vi "Gasteiler Korrektur.vi"() -> ()   [LabVIEW 2020, in "Linearisierung v2.lvlib" / "Gasteiler.lvlib"]
uses:
  Gasteiler.lvlib
  Visualisierungs Elemente/Button.ctl
  Aktion FGV Gasteiler Korrektur.ctl
  Allgemein/allgemeine Sub-VIs.lvlib
panel:
  in  "Aktiv":bool
  out "Gültig":bool
  in  "Gültigkeit bis":timestamp[](array[timestamp]) format="%<%Y/%m/%d>T"
  in  "Gasteiler":enum16{"1", "2", "3", "4", "5"}(ring)
  in  "Seriennummer":string[](array[string])
  in  "Stopp":T1
  in  "Speichern":T1
  in  "Abweichung":sgl[][](array[numeric]) format="%#_5g"
  # "Gasteiler Abweichung"
  # "100%"
  # "90%"
  # "80%"
  # "70%"
  # "60%"
  # "50%"
  # "40%"
  # "30%"
  # "20%"
  # "10%"
  # "0%"
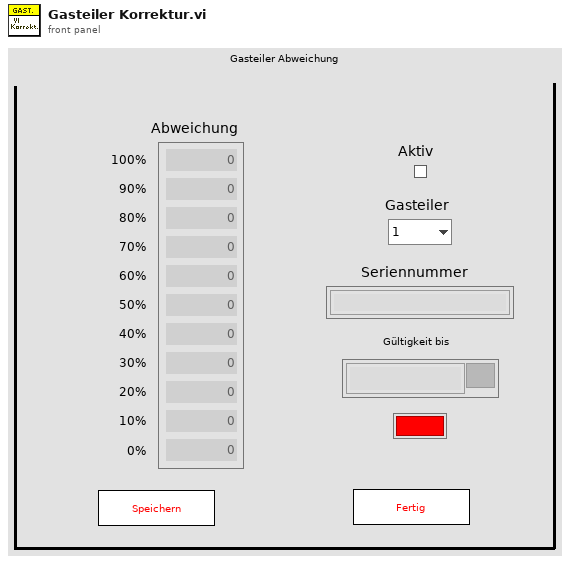
[diagram p1: front panel]
types:
  T1 = typedef "Button.ctl" = bool
  T2 = typedef "Linearisierung v2.lvlib/Gasteiler.lvlib/Aktion FGV Gasteiler Korrektur.ctl" = enum16{"lesen", "schreiben", "laden", "speichern", "B-nr und Gültig", "Gasteilernr.", "Vereinzeln", "aktiv"}
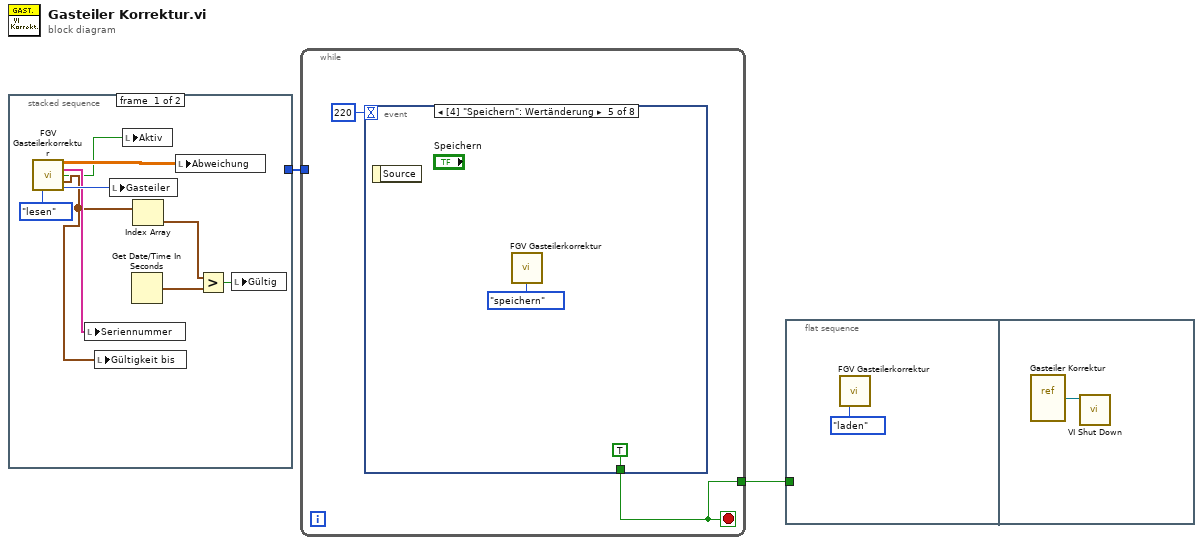
[diagram p0: block diagram]
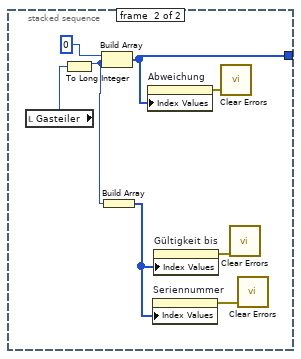
[diagram p2: hidden frame]
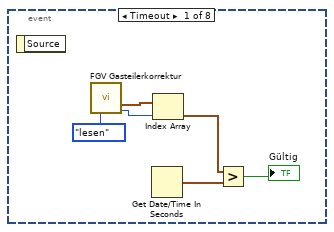
[diagram p3: hidden frame]
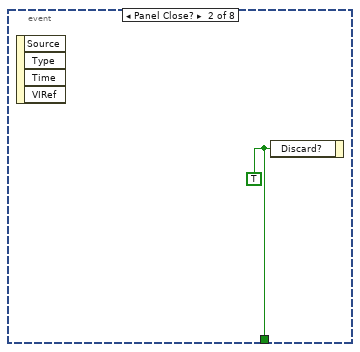
[diagram p4: hidden frame]
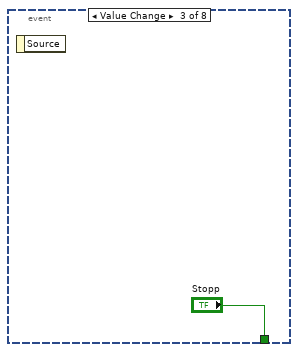
[diagram p5: hidden frame]
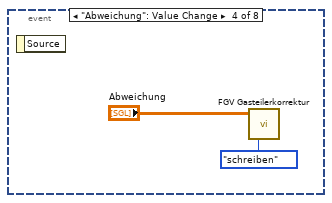
[diagram p6: hidden frame]
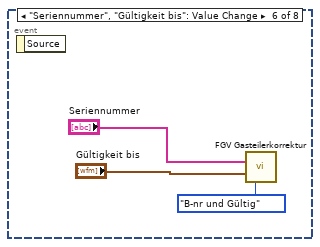
[diagram p7: hidden frame]
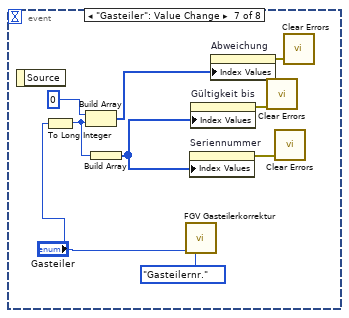
[diagram p8: hidden frame]
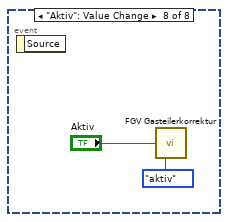
[diagram p9: hidden frame]
diagram:
  n1 = stacked-sequence {
    tunnel: [_ w16] -> w1
    frame #0 {
      n2 = call "FGV Gasteilerkorrektur.vi"("Aktion"=Aktion_FGV_Gasteiler_Korrektur."lesen") -> ("Abweichung"=w8:sgl[][], "Bevesnummer"=w9:string[], "Aktiv"=w3:bool, "Gültigkeit bis"=w5:timestamp[], "Gasteiler"=w10:enum16{"1", "2"})  [unwired: 9 in, 1 out]
      n3 = local write "Seriennummer"(w9) -> ()
      n4 = local write "Gültigkeit bis"(w5) -> ()
      n5 = local write "Gasteiler"(w10) -> ()
      n6 = local write "Aktiv"(w3) -> ()
      n7 = Get Date/Time In Seconds() -> (seconds since 1Jan1904=w6:timestamp)
      n8 = Index Array(array=w5) -> (element=w7:timestamp)  [unwired: 1 in]
      n9 = local write "Abweichung"(w8) -> ()
      n10 = Greater?(x=w7, y=w6) -> (0:w4:bool)
      n11 = local write "Gültig"(w4) -> ()
    }
    frame #1 {
      n12 = local read "Gasteiler"() -> (w15:enum16{"1", "2", "3", "4", "5"})
      n13 = To Long Integer(number=w15) -> (32bit integer=w13:i32)
      n14 = Build Array(0, w13) -> (w16:i32[])
      n15 = Build Array(w13) -> (w12:i32[])
      n16 = property on="Abweichung" class="Arr (strikt)"("Index Values"=w16) -> (error out=w17:errorcluster)  [unwired: 2 in, 1 out]
      n17 = property on="Seriennummer" class="Arr (strikt)"("Index Values"=w12) -> (error out=w18:errorcluster)  [unwired: 2 in, 1 out]
      n18 = property on="Gültigkeit bis" class="Arr (strikt)"("Index Values"=w12) -> (error out=w19:errorcluster)  [unwired: 2 in, 1 out]
      n19 = call <vilib>:"Clear Errors.vi"("error in (no error)"=w17) -> ()  [unwired: 5 in, 2 out]
      n20 = call <vilib>:"Clear Errors.vi"("error in (no error)"=w19) -> ()  [unwired: 5 in, 2 out]
      n21 = call <vilib>:"Clear Errors.vi"("error in (no error)"=w18) -> ()  [unwired: 5 in, 2 out]
    }
  }
  n22 = while {
    tunnel: [w20] -> w2
    tunnel: w1 -> [_]
    stop <- w20 stop-if-true
    n23 = event shown="[4] \"Speichern\": Wertänderung" {
      selector: _ -> [_ _ _ _ _ _ _ _]
      dyn-events: _ -> [_ _ _ _ _ _ _ _]
      timeout: 220 -> [_ _ _ _ _ _ _ _]
      tunnel: [_ w28 "Stopp" _ T1 TRUE ("Stopp") _ _ _] -> w20
      event Timeout {
        n24 = event-data() -> ()  [unwired: 1 in, 1 out]
        n25 = call "FGV Gasteilerkorrektur.vi"("Aktion"=Aktion_FGV_Gasteiler_Korrektur."lesen") -> ("Gültigkeit bis"=w26:timestamp[], "Gasteiler"=w22:enum16{"1", "2"})  [unwired: 9 in, 4 out]
        n26 = Get Date/Time In Seconds() -> (seconds since 1Jan1904=w25:timestamp)
        n27 = Index Array(array=w26, index=w22) -> (element=w24:timestamp)
        n28 = Greater?(x=w24, y=w25) -> (0:→"Gültig":bool)
      }
      event Panel Close? {
        w28 = TRUE ("Verwerfen?")
        n29 = event-data() -> ()  [unwired: 1 in, 4 out]
        n30 = event-data("Discard?"=w28) -> ()  [unwired: 1 in, 1 out]
      }
      event Value Change {
        n31 = event-data() -> ()  [unwired: 1 in, 1 out]
      }
      event "Abweichung": Value Change {
        n32 = event-data() -> ()  [unwired: 1 in, 1 out]
        n33 = call "FGV Gasteilerkorrektur.vi"("Abweichung"="Abweichung", "Aktion"=Aktion_FGV_Gasteiler_Korrektur."schreiben") -> ()  [unwired: 8 in, 6 out]
      }
      event Value Change {
        n34 = event-data() -> ()  [unwired: 1 in, 1 out]
        n35 = call "FGV Gasteilerkorrektur.vi"("Aktion"=Aktion_FGV_Gasteiler_Korrektur."speichern") -> ()  [unwired: 9 in, 6 out]
      }
      event "Seriennummer", "Gültigkeit bis": Value Change {
        n36 = event-data() -> ()  [unwired: 1 in, 1 out]
        n37 = call "FGV Gasteilerkorrektur.vi"("Bevesnummer"="Seriennummer", "Gültigkeit bis"="Gültigkeit bis", "Aktion"=Aktion_FGV_Gasteiler_Korrektur."B-nr und Gültig") -> ()  [unwired: 7 in, 6 out]
      }
      event "Gasteiler": Value Change {
        n38 = event-data() -> ()  [unwired: 1 in, 1 out]
        n39 = To Long Integer(number="Gasteiler") -> (32bit integer=w38:i32)
        n40 = Build Array(0, w38) -> (w41:i32[])
        n41 = Build Array(w38) -> (w37:i32[])
        n42 = call "FGV Gasteilerkorrektur.vi"("Gasteiler"="Gasteiler", "Aktion"=Aktion_FGV_Gasteiler_Korrektur."Gasteilernr.") -> ()  [unwired: 8 in, 6 out]
        n43 = property on="Seriennummer" class="Arr (strikt)"("Index Values"=w37) -> (error out=w44:errorcluster)  [unwired: 2 in, 1 out]
        n44 = property on="Gültigkeit bis" class="Arr (strikt)"("Index Values"=w37) -> (error out=w43:errorcluster)  [unwired: 2 in, 1 out]
        n45 = property on="Abweichung" class="Arr (strikt)"("Index Values"=w41) -> (error out=w42:errorcluster)  [unwired: 2 in, 1 out]
        n46 = call <vilib>:"Clear Errors.vi"("error in (no error)"=w43) -> ()  [unwired: 5 in, 2 out]
        n47 = call <vilib>:"Clear Errors.vi"("error in (no error)"=w44) -> ()  [unwired: 5 in, 2 out]
        n48 = call <vilib>:"Clear Errors.vi"("error in (no error)"=w42) -> ()  [unwired: 5 in, 2 out]
      }
      event "Aktiv": Value Change {
        n49 = event-data() -> ()  [unwired: 1 in, 1 out]
        n50 = call "FGV Gasteilerkorrektur.vi"("Aktiv"="Aktiv", "Aktion"=Aktion_FGV_Gasteiler_Korrektur."aktiv") -> ()  [unwired: 8 in, 6 out]
      }
    }
  }
  n51 = flat-sequence {
    tunnel: w2 -> [_]
    frame #0 {
      n52 = call "FGV Gasteilerkorrektur.vi"("Aktion"=Aktion_FGV_Gasteiler_Korrektur."laden") -> ()  [unwired: 9 in, 6 out]
    }
    frame #1 {
      n53 = vi-ref "Gasteiler Korrektur.vi"() -> (w49:refnum<vi>)
      n54 = call "VI Shut Down.vi"("VI Referenz"=w49) -> ()  [unwired: 11 in]
    }
  }
